vi "Point in Polygon_Main.vi"(6 "tolerance":dbl=1e-09, 8 "Polygon Y":dbl[](array[numeric]), 9 "Polygon X":dbl[](array[numeric]), 10 "y":dbl, 11 "x":dbl) -> (3 "position":T1 items=["Inside", "On Boundary", "Outside"])   [LabVIEW 2020, in "NI_AAL_Geometry.lvlib"]
uses:
  <vilib>/Analysis/NI_AAL_Geometry.lvlib
  <vilib>/Analysis/geometry.llb/Point in Polygon Position.ctl
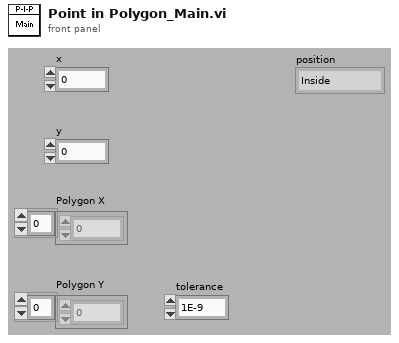
[diagram p1: front panel]
types:
  T1 = typedef "NI_AAL_Geometry.lvlib/Point in Polygon Position.ctl" = u16
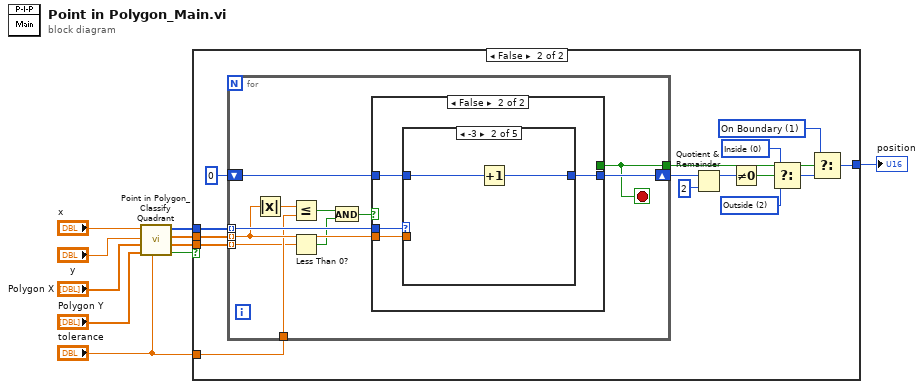
[diagram p0: block diagram]
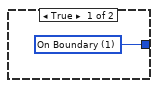
[diagram p2: hidden frame]
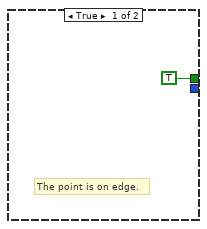
[diagram p3: hidden frame]
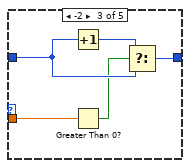
[diagram p5: hidden frame]
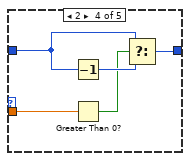
[diagram p6: hidden frame]
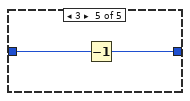
[diagram p7: hidden frame]
diagram:
  n1 = call <vilib>:"Point in Polygon_Classify Quadrant.vi"("tolerance"="tolerance", "Polygon Y"="Polygon Y", "Polygon X"="Polygon X", "y"="y", "x"="x") -> ("vertex?"=w3:bool, "Edge Angle"=w2:dbl[], "Edge Direct"=w9:dbl[], "Edge Quad"=w10:i16[])  [unwired: 3 in]
  n2 = case shown="False" w3 {
    tunnel: w10 -> [_ w21]
    tunnel: [w11 w14] -> w4
    tunnel: w9 -> [_ w22]
    tunnel: w2 -> [_ w13]
    tunnel: "tolerance" -> [_ w12]
    frame True {
      w11 = T1 1 items=["Inside", "On Boundary", "Outside"] ("position")
    }
    frame False {
      w16 = T1 1 items=["Inside", "On Boundary", "Outside"] ("position")
      w18 = T1 2 items=["Inside", "On Boundary", "Outside"] ("position")
      w19 = T1 0 items=["Inside", "On Boundary", "Outside"] ("position")
      n3 = for {
        tunnel: w21 -> [w37] mode=indexing
        shift-right: [w35] -> w23
        shift-left: 0 -> [w36]
        tunnel: w22 -> [w33] mode=indexing
        tunnel: [w34] -> w17
        tunnel: w13 -> [w31] mode=indexing
        tunnel: w12 -> [w32]
        stop <- w34 stop-if-true
        n4 = Absolute Value(x=w33) -> (abs(x)=w27:dbl)
        n5 = Less Or Equal?(x=w27, y=w32) -> (x <= y?=w30:bool)
        n6 = Less Than 0?(x=w31) -> (x < 0?=w29:bool)
        n7 = And(x=w30, y=w29) -> (x .and. y?=w28:bool)
        n8 = case shown="False" w28 {
          tunnel: w37 -> [_ w42]
          tunnel: w36 -> [_ w41]
          tunnel: [_ w40] -> w35
          tunnel: [TRUE _] -> w34
          tunnel: w33 -> [_ w39]
          frame True {
            # "The point is on edge."
          }
          frame False {
            n9 = case shown="-3" w42 {
              tunnel: w41 -> [w43 w44 w50 w54 w56]
              tunnel: [w43 w45 w49 w55 w57] -> w40
              tunnel: w39 -> [_ _ w48 w53 _]
              frame 0, Default {
              }
              frame -3 {
                n10 = Increment(x=w44) -> (x+1=w45:i32)
              }
              frame -2 {
                n11 = Increment(x=w50) -> (x+1=w47:i32)
                n12 = Greater Than 0?(x=w48) -> (x > 0?=w46:bool)
                n13 = Select(t=w47, s=w46, f=w50) -> (s? t:f=w49:i32)
              }
              frame 2 {
                n14 = Decrement(x=w54) -> (x-1=w52:i32)
                n15 = Greater Than 0?(x=w53) -> (x > 0?=w51:bool)
                n16 = Select(t=w54, s=w51, f=w52) -> (s? t:f=w55:i32)
              }
              frame 3 {
                n17 = Decrement(x=w56) -> (x-1=w57:i32)
              }
            }
          }
        }
      }
      n18 = Quotient & Remainder(x=w23, y=2) -> (x-y*floor(x/y)=w24:i32)  [unwired: 1 out]
      n19 = Not Equal To 0?(x=w24) -> (x != 0?=w20:bool)
      n20 = Select(t=w19, s=w20, f=w18) -> (s? t:f=w15:T1)
      n21 = Select(t=w16, s=w17, f=w15) -> (s? t:f=w14:T1)
    }
  }
  "position" <- w4
